vi "Save Fundamental.vi"(8 "error in (no error)":errorcluster, 10 "String":string, 11 "Fundamental-Response":T1={"frequency [Hz]"=[200.0, 212.0, 224.0, 236.0, 250.0, 265.0, 280.0, 300.0, 315.0, 335.0, 355.0, 375.0, 400.0, 425.0, 450.0, 475.0, 500.0, 530.0, 560.0, 600.0, 630.0, 670.0, 710.0, 750.0, 800.0, 850.0, 900.0, 950.0, 1000.0, 1060.0, 1120.0, 1180.0, 1250.0, 1320.0, 1400.0, 1500.0, 1600.0, 1700.0, 1800.0, 1900.0, 2000.0, 2120.0, 2240.0, 2360.0, 2500.0, 2650.0, 2800.0, 3000.0, 3150.0, 3350.0, 3550.0, 3750.0, 4000.0, 4250.0, 4500.0, 4750.0, 5000.0, 5300.0, 5600.0, 6000.0, 6300.0, 6700.0, 7100.0, 7500.0, 8000.0], "amplitude"=[0.08373383766643802, 0.08720256653165395, 0.10216299909051983, 0.12257328841138687, 0.09799617363521568, 0.09308999331866714, 0.09255760054344195, 0.06144947320468093, 0.09799345576034682, 0.08601899423583147, 0.08735366153079059, 0.08566524933231183, 0.06652422278887843, 0.1020328621385577, 0.10143432688172244, 0.09928770099474234, 0.09381790858423543, 0.09045617594098058, 0.09948710909656786, 0.10523182957023507, 0.09022852870341927, 0.06600877030406832, 0.06744144709426814, 0.0763289145732647, 0.08080935378438643, 0.08728241238242278, 0.08127815647631875, 0.09046363263225381, 0.09902477903345173, 0.09475334386154104, 0.09677319912982299, 0.10329477846216732, 0.10283778506980566, 0.09270572918509108, 0.09074263628924208, 0.0971294371970155, 0.09770265947930772, 0.09820932946337788, 0.10409242767991532, 0.09604944256553502, 0.09341298984882208, 0.09434143289735775, 0.07759066500995275, 0.07058477895547258, 0.10024808480334779, 0.0961056829377728, 0.09178264851844328, 0.091526011389544, 0.09680854977268145, 0.10398242444193603, 0.10503762416280657, 0.10023202653569101, 0.10732936877596516, 0.12137499244376211, 0.1273951297534099, 0.1294428153022033, 0.13157459738545074, 0.1258042595931751, 0.11576656465103383, 0.10651128057141616, 0.11298962916691604, 0.12072532203570616, 0.13717741081625343, 0.14691078493762416, 0.17768222272226997]}) -> (0 "error out":errorcluster)   [LabVIEW 2018]
uses:
  <vilib>/Utility/file.llb/Write Delimited Spreadsheet (string).vi
panel:
  out "Array":string[][](array[string])
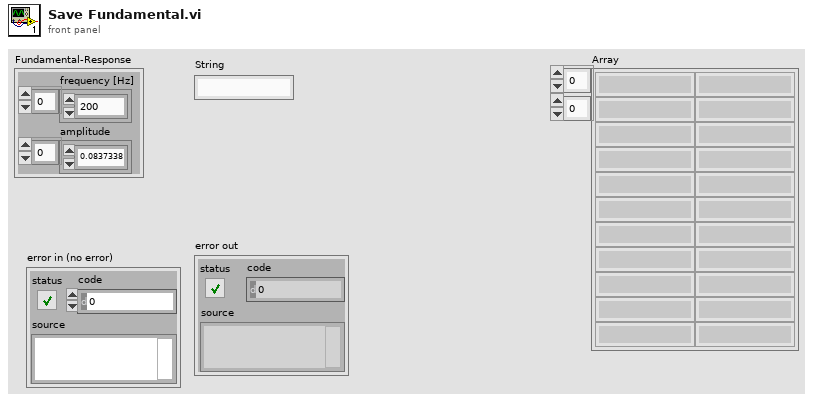
[diagram p1: front panel]
types:
  T1 = cluster{"frequency [Hz]":dbl[], "amplitude":dbl[]}
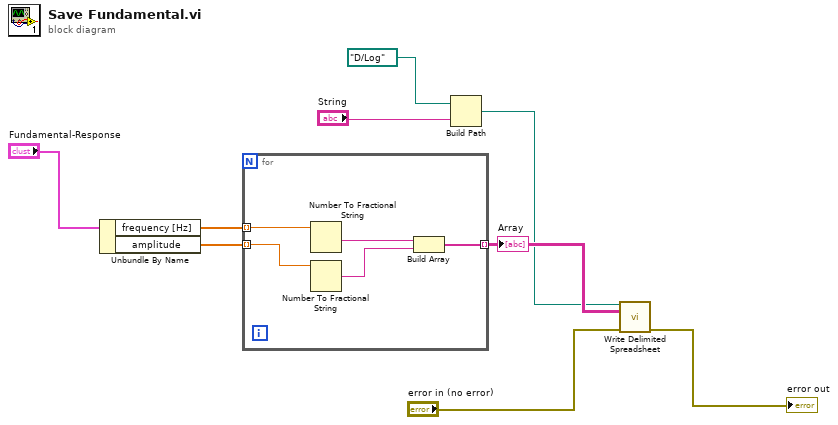
[diagram p0: block diagram]
diagram:
  n1 = Unbundle By Name("Fundamental-Response") -> ("frequency [Hz]"=w8:dbl[], "amplitude"=w7:dbl[])
  n2 = for {
    tunnel: w8 -> [w14] mode=indexing
    tunnel: w7 -> [w13] mode=indexing
    tunnel: [w10] -> w6 mode=indexing
    n3 = Number To Fractional String(number=w14) -> (F-format string=w12:string)  [unwired: 3 in]
    n4 = Number To Fractional String(number=w13) -> (F-format string=w11:string)  [unwired: 3 in]
    n5 = Build Array(w12, w11) -> (w10:string[])
  }
  "Array" <- w6
  n6 = Build Path(base path=path "D:/Log" ("file path (dialog if empty)"), name or relative path="String") -> (appended path=w1:path)
  n7 = call-poly <vilib>:"Write Delimited Spreadsheet.vi"("file path (dialog if empty)"=w1, "2D data"=w6, "error in (no error)"="error in (no error)") -> ("error out"=→"error out":errorcluster)  [unwired: 11 in, 1 out]
